vi "Analyse-scan-file.vi"(8 "error in (no error)":errorcluster, 11 "Object ref in":T1) -> (0 "error out":errorcluster, 3 "Object ref out":T1)   [LabVIEW 2013, in "MaterialCharacterization.lvlib" / "MC-Main.lvclass"]
uses:
  MC-Main.lvclass
  Object-reference.ctl
  MC-Main.lvclass/MC-Main.ctl
  Read Parser.vi
  ScanParser/MC-ScanParser.lvclass
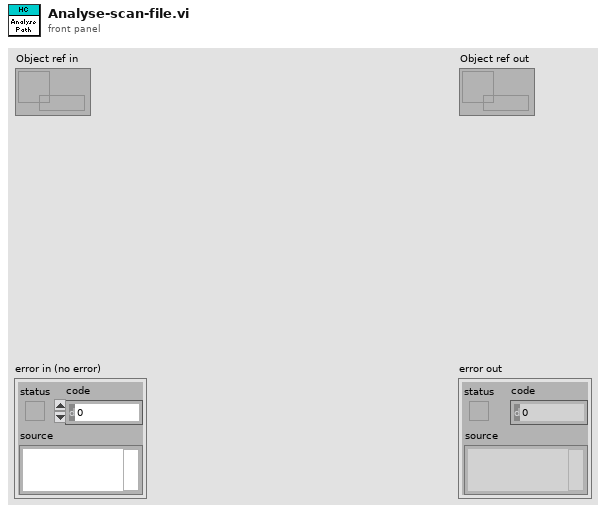
[diagram p1: front panel]
types:
  T1 = typedef "MaterialCharacterization.lvlib/MC-Main.lvclass/Object-reference.ctl" = refnum<data-value>
  T2 = typedef "MaterialCharacterization.lvlib/MC-ScanParser.lvclass/Object-reference.ctl" = refnum<data-value>
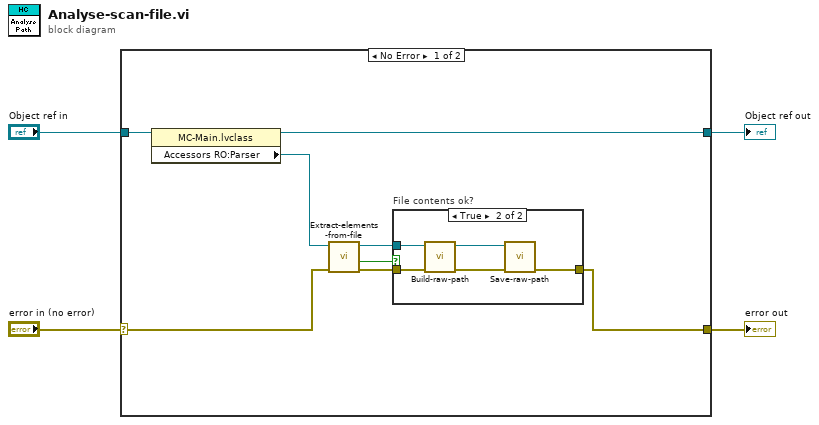
[diagram p0: block diagram]
diagram:
  n1 = case shown="No Error" "error in (no error)" {
    selector: "error in (no error)" -> [w6 w20]
    tunnel: [w5 w20] -> w3
    tunnel: [w11 w19] -> w1
    tunnel: "Object ref in" -> [w12 w19]
    frame No Error {
      n2 = property class="MC-Main.lvclass"(reference=w12) -> (reference out=w11:T1, "Accessors RO:Parser"=w10:T2)  [unwired: 1 in, 1 out]
      n3 = call "Extract-elements-from-file.vi"("error in (no error)"=w6, "Reference in"=w10) -> ("error out"=w7:errorcluster, "Succes?"=w8:bool, "Reference out"=w9:T2)  [unwired: 7 in]
      n4 = case "File contents ok?" shown="True" w8 {
        tunnel: w9 -> [_ w18]
        tunnel: w7 -> [w13 w17]
        tunnel: [w13 w15] -> w5
        frame False {
        }
        frame True {
          n5 = call "Build-raw-path.vi"("error in (no error)"=w17, "Reference in"=w18) -> ("error out"=w16:errorcluster, "Reference out"=w14:T2)  [unwired: 7 in, 1 out]
          n6 = call "Save-raw-path.vi"("error in (no error)"=w16, "Reference in"=w14) -> ("error out"=w15:errorcluster)  [unwired: 8 in, 1 out]
        }
      }
    }
    frame Error {
    }
  }
  "error out" <- w3
  "Object ref out" <- w1
